vi "CoinDetector2 - コピー (2).vi"() -> ()   [LabVIEW 2020]
panel:
  in  "Start":bool
  out "Now Freq":dbl
  in  "stop":bool
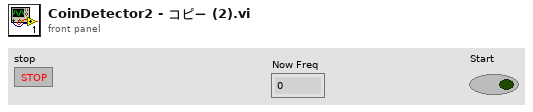
[diagram p1: front panel]
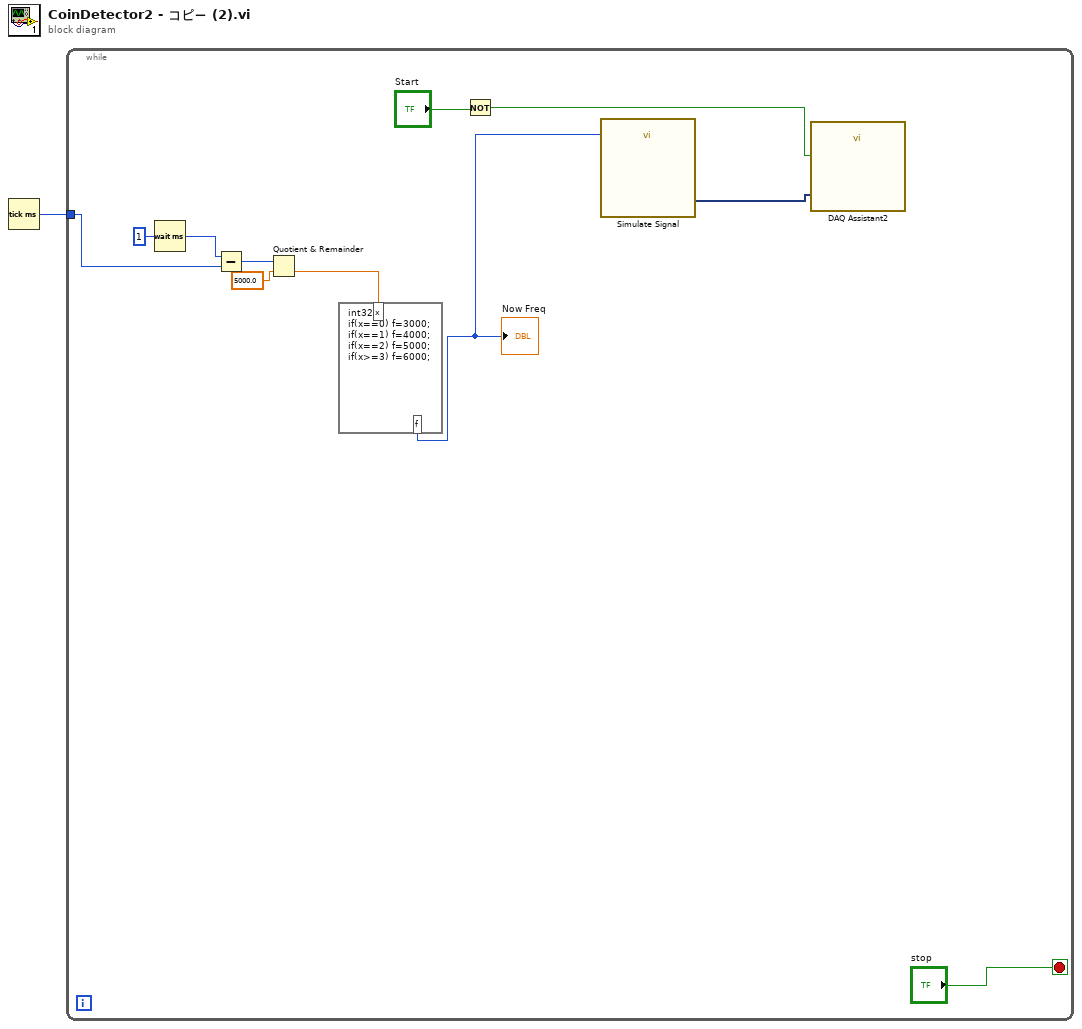
[diagram p0: block diagram]
diagram:
  n1 = Tick Count (ms)() -> (millisecond timer value=w1:u32)
  n2 = while {
    tunnel: w1 -> [w2]
    stop <- "stop" stop-if-true
    n3 = Wait (ms)(milliseconds to wait=u32 1) -> (millisecond timer value=w6:u32)
    n4 = Subtract(x=w6, y=w2) -> (x-y=w7:u32)
    n5 = Quotient & Remainder(x=w7, y=5000.0) -> (floor(x/y)=w8:dbl)  [unwired: 1 out]
    n6 = formula code="int32 f;\nif(x==0) f=3000;\nif(x==1) f=4000;\nif(x==2) f=5000;\nif(x>=3) f=6000;"("x"=w8) -> ("f"=w9:i32)
    "Now Freq" <- w9
    n7 = Not(x="Start") -> (.not. x?=w11:bool)
    n8 = call "Simulate Signal"("Frequency"=w9) -> ("Sine"=w5:dynamicdata)  [unwired: 13 in, 1 out]
    n9 = call "DAQ Assistant2"("data"=w5, "stop (F)"=w11) -> ()  [unwired: 15 in, 3 out]
  }
